vi "Global_Device(SubVI).vi"(10 "Device in":string, 11 "R/W":T1) -> (2 "Device out":string)   [LabVIEW 2015]
uses:
  R_W.ctl
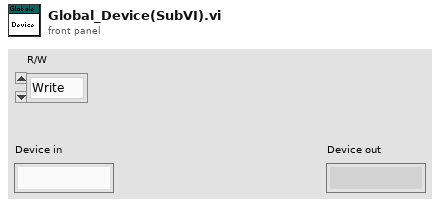
[diagram p1: front panel]
types:
  T1 = typedef "R_W.ctl" = enum16{"Write", "Read", "RAZ"}
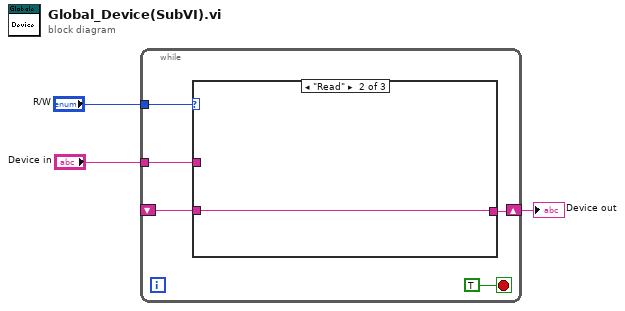
[diagram p0: block diagram]
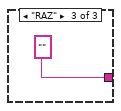
[diagram p3: hidden frame]
diagram:
  n1 = while {
    tunnel: "R/W" -> [w8]
    shift-right: [w6] -> w1
    shift-left: _ -> [w5]
    tunnel: "Device in" -> [w4]
    stop <- TRUE stop-if-true
    n2 = case shown="\"Read\"" w8 {
      tunnel: [w9 w10 ""] -> w6
      tunnel: w5 -> [_ w10 _]
      tunnel: w4 -> [w9 _ _]
      frame "Write", Default {
      }
      frame "Read" {
      }
      frame "RAZ" {
      }
    }
  }
  "Device out" <- w1
